vi "LoadSavedQueueList.vi"(0 "Program Interface in":refnum<class "Program Interface.lvclass">, 5 "error in (no error)":errorcluster) -> (14 "Program Interface out":refnum<class "Program Interface.lvclass">, 19 "error out":errorcluster)   [LabVIEW 2019, in "Program Interface.lvclass"]
uses:
  Program Interface.lvclass
  Program Interface.lvclass/Program Interface.ctl
  SavedQueue.ctl
  <vilib>/Utility/file.llb/Read Delimited Spreadsheet (string).vi
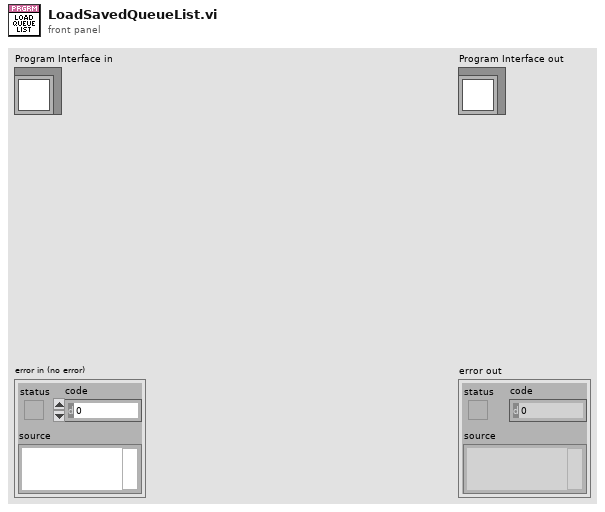
[diagram p1: front panel]
types:
  T1 = typedef "Program Interface.lvclass/SavedQueue.ctl" = cluster{"Name":string, "Programs":string[]}
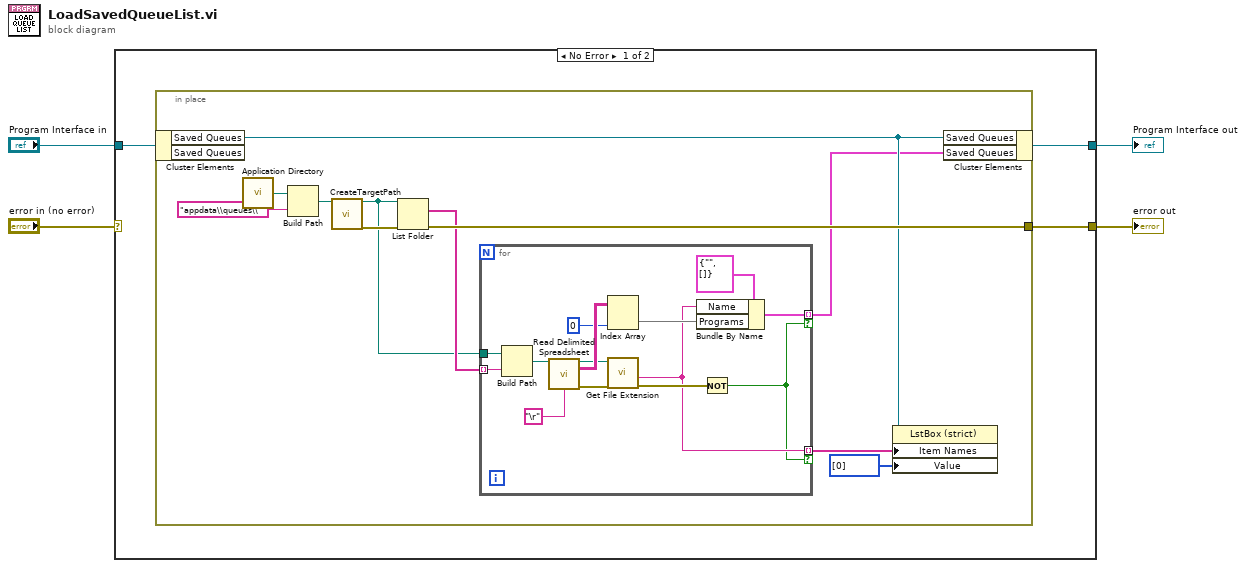
[diagram p0: block diagram]
diagram:
  n1 = case shown="No Error" "error in (no error)" {
    selector: "error in (no error)" -> [_ w34]
    tunnel: [w7 w34] -> w3
    tunnel: [w5 w33] -> w1
    tunnel: "Program Interface in" -> [w6 w33]
    frame No Error {
      n2 = in-place {
        in-place-border: [w14] -> w7
        n3 = in-place-cluster #1(w6) -> ("Saved Queues"=w10:refnum<vi>)  [unwired: 1 out]
        n4 = call <vilib>:"Application Directory.vi"() -> ("Application Directory"=w18:path)
        n5 = Build Path(base path=w18, name or relative path="appdata\\queues\\") -> (appended path=w16:path)
        n6 = call "CreateTargetPath.vi"("Target Path In"=w16) -> ("Target Path Out"=w12:path, "Error Out"=w15:errorcluster)  [unwired: 17 in]
        n7 = List Folder(path=w12, error in=w15) -> (filenames=w13:string[], error out=w14:errorcluster)  [unwired: 2 in, 2 out]
        n8 = for {
          tunnel: w13 -> [w30] mode=indexing
          tunnel: w12 -> [w31]
          tunnel: [w22] -> w8 mode=indexing if=w19
          tunnel: [w20] -> w9 mode=indexing if=w19
          n9 = Build Path(base path=w31, name or relative path=w30) -> (appended path=w29:path)
          n10 = call-poly <vilib>:"Read Delimited Spreadsheet.vi"("file path (dialog if empty)"=w29, "delimiter (\\t)"="\r" ("delimiter (\\t)")) -> ("new file path (Not A Path if cancelled)"=w25:path, "all rows"=w28:string[][], "error out"=w24:errorcluster)  [unwired: 8 in, 3 out]
          n11 = Index Array(array=w28, index (col)=0 ("disabled index (col)")) -> (element=w23:string[])  [unwired: 1 in]
          n12 = call <vilib>:"Get File Extension.vi"("error in (no error)"=w24, "file"=w25) -> ("error out"=w21:errorcluster, "filename without extension"=w20:string)  [unwired: 5 in, 3 out]
          n13 = Bundle By Name(cluster=T1 {"Name"="", "Programs"=[]} ("Saved Queue"), "Name"=w20, "Programs"=w23) -> (w22:T1)
          n14 = Not(x=w21) -> (.not. x?=w19:bool)
        }
        n15 = property class="LstBox (strict)"(reference=w10, "Item Names"=w9, "Value"=i32[] [0]) -> ()  [unwired: 1 in, 2 out]
        n16 = in-place-cluster #1("Saved Queues"=w10, "Saved Queues"=w8) -> (w5:refnum<class "Program Interface.lvclass">)
      }
    }
    frame Error {
    }
  }
  "error out" <- w3
  "Program Interface out" <- w1
